vi "Initialize.vi"(7 "App Reference (This Application)":refnum<vi>, 8 "error in (no error)":errorcluster {"code" format="Error %.0f"}, 10 "Settings Path":path, 11 "UI Interaction":refnum<class "UI Interaction.lvclass">) -> (0 "error out":errorcluster {"code" format="Error %.0f"}, 3 "VIDoc Parser Out":refnum<class "VIDoc Parser.lvclass">)   [LabVIEW 2023, in "VIDoc Parsing.lvlib" / "VIDoc Parser.lvclass"]
uses:
  VIDoc Parser.lvclass
  UI Interaction/UI Interaction.lvclass
  VIDoc Parser.lvclass/VIDoc Parser.ctl
  Settings/Parser Settings/Parser Settings.lvclass
  Settings/Printer Settings/Printer Settings.lvclass
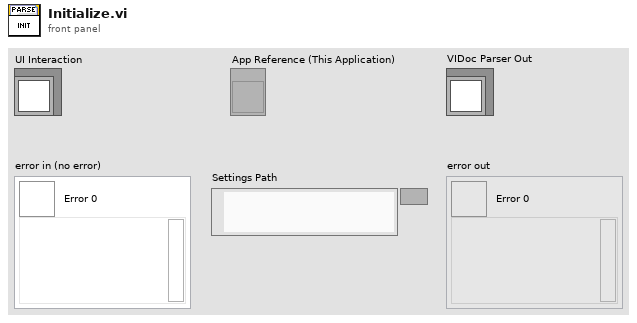
[diagram p1: front panel]
types:
  T1 = typedef "VIDoc Parsing.lvlib/Parser Settings.lvclass/Parser Settings Cluster.ctl" = cluster{"Draw Controls":T2, "Max Control Recursion Depth":i32, "UI Bookmarks":string[], "Subpanel Bookmarks":string[], "Dialog Bookmarks":string[]}
  T2 = typedef "VIDoc Parsing.lvlib/Parser Settings.lvclass/Draw Controls Cluster.ctl" = cluster{"Subpanels":bool, "Tabs":bool, "TypeDefs":bool, "Error Clusters":T3, "DVRs":T3, "Queues & Notifiers":T3}
  T3 = typedef "VIDoc Parsing.lvlib/Parser Settings.lvclass/Draw Option Enum.ctl" = enum16{"Ignore", "Draw", "Draw + Contents"}
  T4 = typedef "VIDoc Printer.lvlib/Printer Settings.lvclass/Enabled Sections Cluster.ctl" = cluster{"Projects":bool, "User Interfaces":bool, "Subpanels":bool, "Dialogs":bool, "Interfaces":bool, "Classes":bool, "Libraries":bool, "VIs":bool, "Controls":bool, "LLBs":bool}
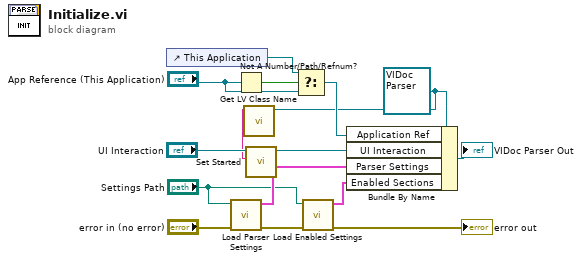
[diagram p0: block diagram]
diagram:
  w2 = refnum<class "VIDoc Parser.lvclass"> refnum ("Fetch Parser out")
  n1 = control-ref of="This Application"() -> (w13:refnum<vi>)
  n2 = call "Load Parser Settings.vi"("Error in"="error in (no error)", "Settings Path"="Settings Path") -> ("Error out"=w8:errorcluster, "Parser Settings"=w9:T1)  [unwired: 7 in, 1 out]
  n3 = Not A Number/Path/Refnum?(number/path/refnum="App Reference (This Application)") -> (NaN/Path/Refnum?=w14:bool)
  n4 = call <vilib>:"Get LV Class Name.vi"("object"=w2) -> ("class name"=w1:string)  [unwired: 9 in, 1 out]
  n5 = call-dynamic "Set Started.vi"("Process"=w1, "UI Interaction in"="UI Interaction") -> ("UI Interaction out"=w3:refnum<class "UI Interaction.lvclass">)  [unwired: 8 in, 1 out]
  n6 = Select(t=w13, s=w14, f="App Reference (This Application)") -> (s? t:f=w11:refnum<vi>)
  n7 = call "Load Enabled Settings.vi"("Error in"=w8, "Settings Path"="Settings Path") -> ("Error out"=→"error out":errorcluster, "Enabled Sections"=w5:T4)  [unwired: 7 in, 1 out]
  n8 = Bundle By Name(cluster=w2, "Application Ref"=w11, "UI Interaction"=w3, "Parser Settings"=w9, "Enabled Sections"=w5) -> (→"VIDoc Parser Out":refnum<class "VIDoc Parser.lvclass">)
